vi "Write Value.vi"(6 "Position":i32, 8 "error in (no error)":errorcluster, 9 "Value":string, 10 "Label":string, 11 "Test Class in":refnum<class "Test Class.lvclass">) -> (0 "error out":errorcluster)   [LabVIEW 2017, in "Test Class.lvclass"]
uses:
  Test Class.lvclass
  <vilib>/TSS/ACRObat Test Framework/Core Launcher/Core Manager Methods -- Enum.ctl
  <vilib>/TSS/ACRObat Test Framework/Core Launcher/Core Launcher.lvlib
  <vilib>/TSS/ACRObat Test Framework/Classes/Data/Data Repo/Class/Data Repo.lvclass
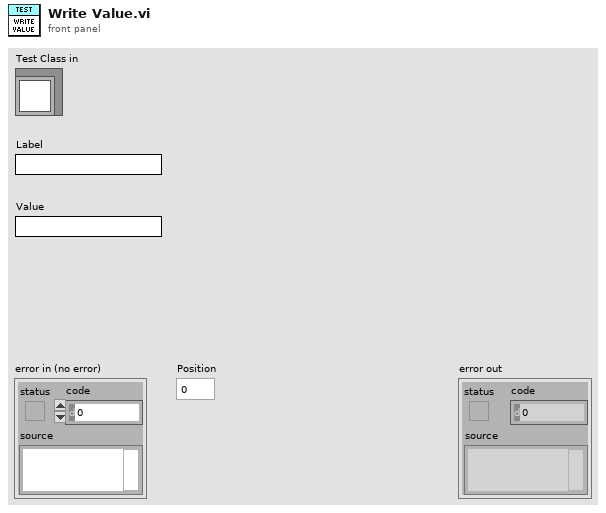
[diagram p1: front panel]
types:
  T1 = typedef "Core Launcher.lvlib/Core Manager Methods -- Enum.ctl" = enum16{"Spawn Objects", "Get Objects", "Destroy Objects"}
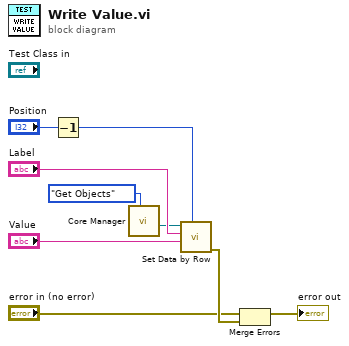
[diagram p0: block diagram]
diagram:
  n1 = Decrement(x="Position") -> (x-1=w3:i32)
  n2 = call <vilib>:"Core Manager.vi"("Method"=Core_Manager_Methods_--_Enum."Get Objects") -> ("Data Repo"=w5:refnum<class "Data Repo.lvclass">)  [unwired: 6 in, 4 out]
  n3 = call <vilib>:"Set Data by Row.vi"("Row"=w3, "Value"="Value", "Header"="Label", "Acrobat Template in"=w5) -> ("error out"=w9:errorcluster)  [unwired: 6 in, 1 out]
  n4 = Merge Errors("error in (no error)", w9) -> (→"error out":errorcluster)
